vi "Inficon Controller - Main.vi"() -> ()   [LabVIEW 2014]
uses:
  Typedef/Inficon - States.ctl
  Typedef/Inficon - Evaporator parameters.ctl
panel:
  in  "Tab Control":T1(tab)
  in  "Reset":bool
  in  "Run process":bool
  in  "Test Connection":bool
  in  "Set parameters":bool
  in  "Final Thickness":dbl caption="Final Thickness [kÅ]" min=0.0 max=999.0 step=0.001 format="%.;%.3f"
  in  "Exit":bool
  in  "Select Material":u16(ring) items=["None", "Al (Alluminio) - Rotazione", "Al (Alluminio) - Fisso", "Ag (Argento) - Fisso", "Au (Oro) - Rotazione", "Au (Oro) - Fisso", "In (Indio) - Rotazione", "In (Indio) - Fisso", "Cr (Cromo) - Rotazione", "Cr (Cromo) - Fisso", "Cu (Rame) - Rotazione", "Cu (Rame) - Fisso", "Costantana (Cu 55% ; Ni 45%) - Fisso", "Ge (Germanio) - Fisso", "Mo (Molibdeno) - Rotazione", "Mo (Molibdeno) - Fisso", "Pd (Palladio) - Fisso"]
  in  "Deposition Rate":dbl caption="Deposition Rate [Å/s]" min=0.0 max=999.9 step=0.1 format="%.;%.1f"
  in  "Max Power":dbl=0.1 min=0.0 max=100.0 step=0.1 format="%.;%.1f"
  out "Thickness":dbl
  out "Dep rate":dbl
  out "Power":dbl
  in  "Generate XML":bool
  in  "Evap params":T2={"Rise Time 1 [mm:ss]"=0.0, "Soak Power 1 [%]"=0.0, "Soak Time 1 [mm:ss]"=0.0, "Rise Time 2 [mm:ss]"=0.0, "Soak Power 2 [%]"=0.0, "Soak Time 2 [mm:ss]"=0.0, "Shutter Delay"=enum."No", "New Rate"=0.0, "Rate Ramp Time [mm:ss]"=0.0, "Idle Ramp [mm:ss]"=0.0, "Idle Power [%]"=0.0, "Time Power"=enum."No", "Xtal Switch S"=0, "Xtal Switch Q"=0, "Tool Factor 1"=10.0, "Tool Factor 2"=10.0, "Deposition Rate [Å/s]"=0.0, "Final Thickness [kÅ]"=0.0, "Thickness Spt [kÅ]"=0.0, "Density [g/cm3]"=0.5, "Z-Ratio"=0.1, "Sensor"=1, "Source"=1, "Crucible"=1, "Control Gain [%]"=0.1, "Control TC [s]"=0.1, "Control DT [s] 2"=0.1, "Max Power"=0.1, "Sample"=1, "Hold Time [mm:ss]"=0.0} caption="Evaporator parameters" {"Hold Time [mm:ss]" min=0.0 max=5999.0 format="%<%M:%S>t"; "Sample" max=99 step=1; "Max Power" min=0.0 max=100.0 step=0.1 format="%.;%.1f"; "Control DT [s] 2" min=0.1 max=100.0 step=0.1 format="%.;%.1f"; "Control TC [s]" min=0.1 max=100.0 step=0.1 format="%.;%.1f"; "Control Gain [%]" min=0.01 max=99.99 step=0.01 format="%.;%.3f"; "Crucible" max=8 step=1; "Source" min=1 max=2 step=1; "Sensor" min=1 max=2 step=1; "Z-Ratio" min=0.1 max=9.999 step=0.001 format="%.;%.3f"; "Density [g/cm3]" min=0.5 max=99.99 step=0.01 format="%.;%.2f"; "Thickness Spt [kÅ]" min=0.0 max=999.0 step=0.001 format="%.;%.3f"; "Final Thickness [kÅ]" min=0.0 max=999.0 step=0.001 format="%.;%.3f"; "Deposition Rate [Å/s]" min=0.0 max=999.9 step=0.1 format="%.;%.1f"; "Tool Factor 2" min=10.0 max=500.0 step=0.1 format="%.;%.1f"; "Tool Factor 1" min=10.0 max=500.0 step=0.1 format="%.;%.1f"; "Xtal Switch Q" max=9 step=1; "Xtal Switch S" max=9 step=1; "Idle Power [%]" min=0.0 max=100.0 step=0.1 format="%.;%.1f"; "Idle Ramp [mm:ss]" min=0.0 max=5999.0 format="%<%M:%S>t"; "Rate Ramp Time [mm:ss]" min=0.0 max=5999.0 format="%<%M:%S>t"; "New Rate" min=0.0 max=999.9 step=0.1 format="%.;%.1f"; "Soak Time 2 [mm:ss]" min=0.0 max=5999.0 format="%<%M:%S>t"; "Soak Power 2 [%]" min=0.0 max=100.0 step=0.1 format="%.;%.1f"; "Soak Time 1 [mm:ss]" min=0.0 max=5999.0 format="%<%M:%S>t"; "Rise Time 2 [mm:ss]" min=0.0 max=5999.0 format="%<%M:%S>t"; "Soak Power 1 [%]" min=0.0 max=100.0 step=0.1 format="%.;%.1f"; "Rise Time 1 [mm:ss]" min=0.0 max=5999.0 format="%<%M:%S>t"}
  in  "Metal name":string
  out "Thickness Plot":dbl(graph)
  out "Dep rate Plot":dbl(graph)
  out "Power Plot":dbl(graph)
  # "Real time monitor"
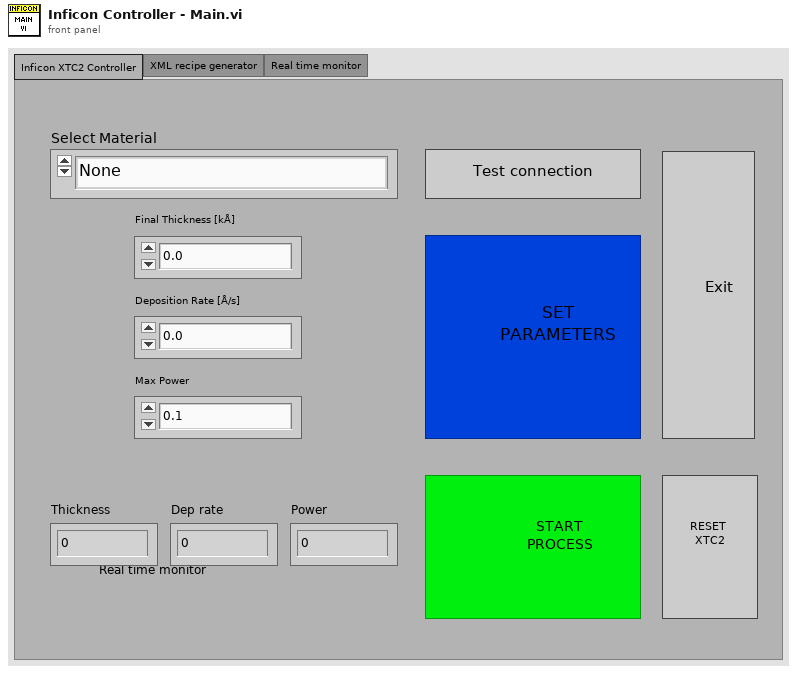
[diagram p1: front panel]
types:
  T1 = enum32{"Inficon XTC2 Controller", "XML recipe generator", "Real time monitor"}
  T2 = typedef "Inficon - Evaporator parameters.ctl" = cluster{"Rise Time 1 [mm:ss]":dbl, "Soak Power 1 [%]":dbl, "Soak Time 1 [mm:ss]":dbl, "Rise Time 2 [mm:ss]":dbl, "Soak Power 2 [%]":dbl, "Soak Time 2 [mm:ss]":dbl, "Shutter Delay":enum16{"No", "Yes"}, "New Rate":dbl, "Rate Ramp Time [mm:ss]":dbl, "Idle Ramp [mm:ss]":dbl, "Idle Power [%]":dbl, "Time Power":enum16{"No", "Yes"}, "Xtal Switch S":u8, "Xtal Switch Q":u8, "Tool Factor 1":dbl, "Tool Factor 2":dbl, "Deposition Rate [Å/s]":dbl, "Final Thickness [kÅ]":dbl, "Thickness Spt [kÅ]":dbl, "Density [g/cm3]":dbl, "Z-Ratio":dbl, "Sensor":u8, "Source":u8, "Crucible":u8, "Control Gain [%]":dbl, "Control TC [s]":dbl, "Control DT [s] 2":dbl, "Max Power":dbl, "Sample":u8, "Hold Time [mm:ss]":dbl}
  T3 = typedef "Inficon - States.ctl" = enum16{"Set Parameters", "Test connection", "Generate XML", "Check for Error", "Set Max Power", "Set Deposition rate", "Read RT parameters", "Start/Stop process", "Reset XTC2", "Exit"}
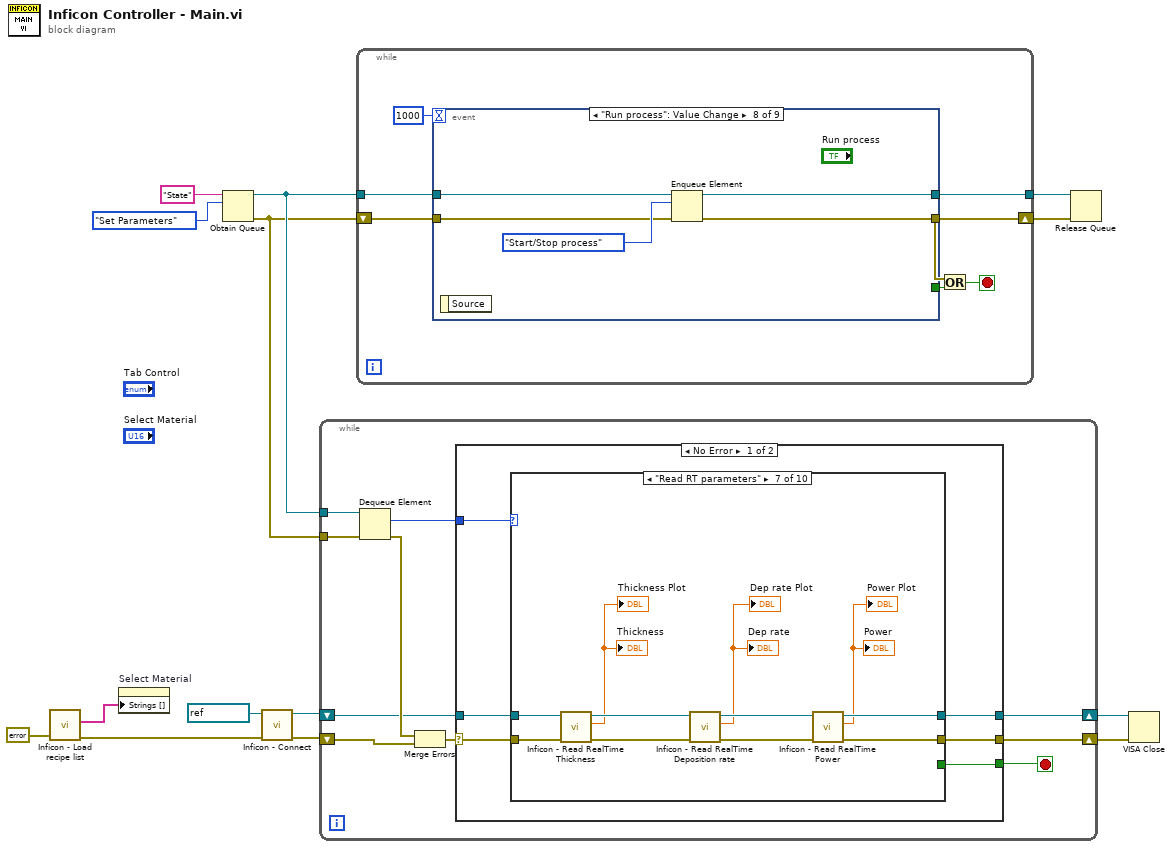
[diagram p0: block diagram]
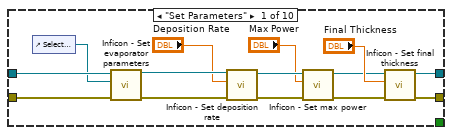
[diagram p2: hidden frame]
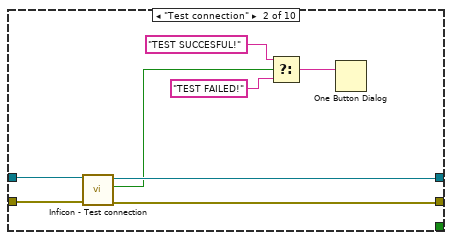
[diagram p3: hidden frame]
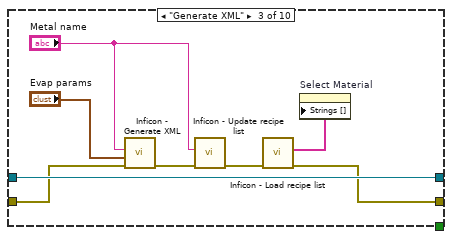
[diagram p4: hidden frame]
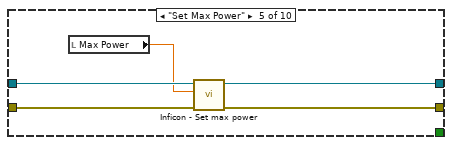
[diagram p6: hidden frame]
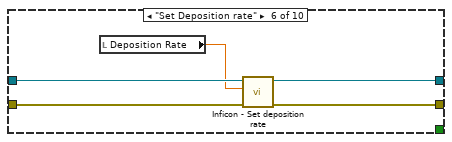
[diagram p7: hidden frame]
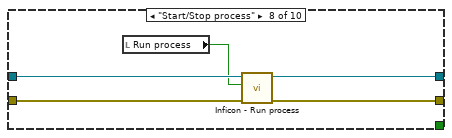
[diagram p8: hidden frame]
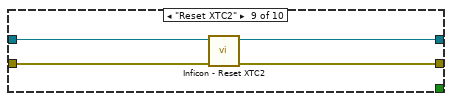
[diagram p9: hidden frame]
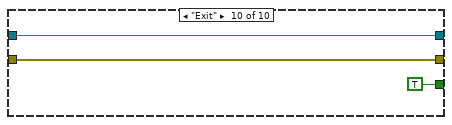
[diagram p10: hidden frame]
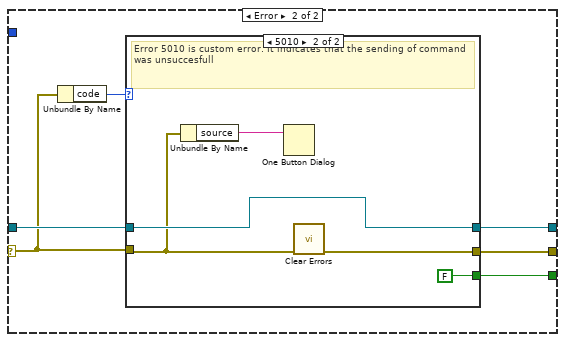
[diagram p11: hidden frame]
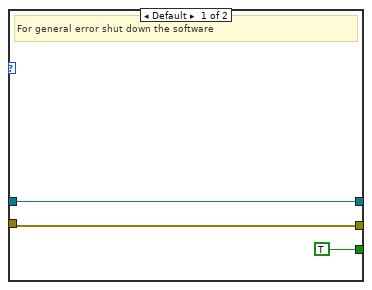
[diagram p12: hidden frame]
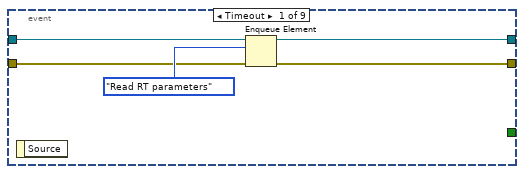
[diagram p13: hidden frame]
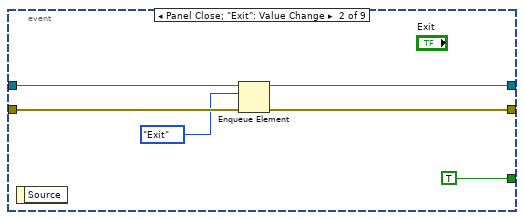
[diagram p14: hidden frame]
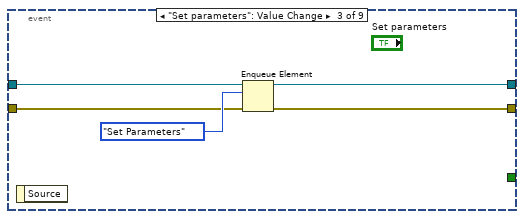
[diagram p15: hidden frame]
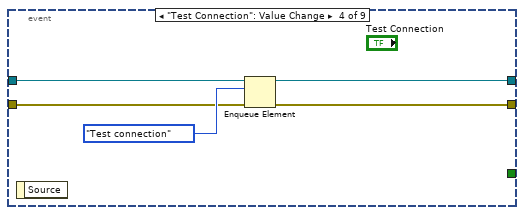
[diagram p16: hidden frame]
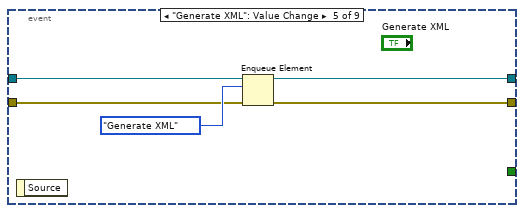
[diagram p17: hidden frame]
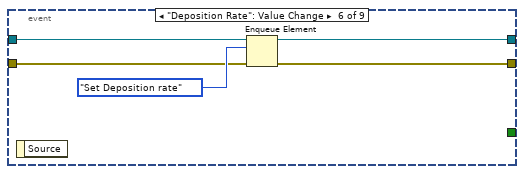
[diagram p18: hidden frame]
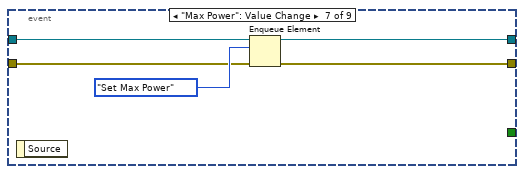
[diagram p19: hidden frame]
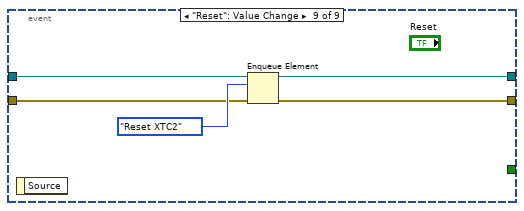
[diagram p20: hidden frame]
diagram:
  n1 = call "Inficon - Load recipe list.vi"("Error In"=errorcluster {"status"=FALSE, "code"=0, "source"=""} ("error out")) -> ("Error Out"=w1:errorcluster, "recipe list"=w5:string[])  [unwired: 9 in]
  n2 = property on="Select Material" class="Ring (strict)"("Strings []"=w5) -> ()  [unwired: 2 in, 2 out]
  n3 = Obtain Queue(name (unnamed)="State", element data type=Inficon_-_States."Set Parameters") -> (queue out=w11:refnum<queue>, error out=w10:errorcluster)  [unwired: 3 in, 1 out]
  n4 = call "Inficon - Connect.vi"("Error In"=w1, "COM in"=refnum<visa-resource-name> "COM5") -> ("Error Out"=w2:errorcluster, "COM out"=w3:refnum<visa-resource-name>)  [unwired: 8 in]
  n5 = while {
    tunnel: w11 -> [w23]
    tunnel: w10 -> [w22]
    shift-right: [w21] -> w8
    shift-left: w2 -> [w19]
    shift-right: [w17] -> w7
    shift-left: w3 -> [w16]
    stop <- w15 stop-if-true
    n6 = Dequeue Element(queue=w23, error in (no error)=w22) -> (element=w24:T3, error out=w18:errorcluster)  [unwired: 1 in, 2 out]
    n7 = Merge Errors(w18, w19) -> (w20:errorcluster)
    n8 = case shown="No Error" w20 {
      selector: w20 -> [w28 w97]
      tunnel: w24 -> [w30 _]
      tunnel: [w25 w100] -> w15
      tunnel: [w29 w96] -> w21
      tunnel: [w27 w99] -> w17
      tunnel: w16 -> [w26 w98]
      frame No Error {
        n9 = case shown="\"Read RT parameters\"" w30 {
          tunnel: [w41 w49 w58 w61 w65 w70 w79 w87 w91 w95] -> w29
          tunnel: w28 -> [w44 w51 w56 w61 w66 w71 w82 w88 w92 w95]
          tunnel: [w42 w50 w60 w62 w64 w69 w76 w85 w89 w94] -> w27
          tunnel: w26 -> [w43 w52 w60 w62 w67 w72 w83 w86 w90 w94]
          tunnel: [_ _ _ _ _ _ _ _ _ TRUE] -> w25
          frame "Set Parameters" {
            n10 = control-ref of="Select Material"() -> (w39:refnum<vi>)
            n11 = call "Inficon - Set evaporator parameters.vi"("Error In"=w44, "Material refnum"=w39, "COM in"=w43) -> ("Error Out"=w33:errorcluster, "COM out"=w38:refnum<visa-resource-name>)  [unwired: 7 in]
            n12 = call "Inficon - Set deposition rate.vi"("Error In"=w33, "Deposition Rate"="Deposition Rate", "COM in"=w38) -> ("Error Out"=w34:errorcluster, "COM out"=w37:refnum<visa-resource-name>)  [unwired: 7 in]
            n13 = call "Inficon - Set max power.vi"("Error In"=w34, "Max Power"="Max Power", "COM in"=w37) -> ("Error Out"=w35:errorcluster, "COM out"=w36:refnum<visa-resource-name>)  [unwired: 7 in]
            n14 = call "Inficon - Set final thickness.vi"("Error In"=w35, "Final Thickness"="Final Thickness", "COM in"=w36) -> ("Error Out"=w41:errorcluster, "COM out"=w42:refnum<visa-resource-name>)  [unwired: 7 in]
          }
          frame "Test connection" {
            n15 = call "Inficon - Test connection.vi"("Error In"=w51, "COM in"=w52) -> ("Error Out"=w49:errorcluster, "Success?"=w48:bool, "COM out"=w50:refnum<visa-resource-name>)  [unwired: 7 in]
            n16 = Select(t="TEST SUCCESFUL!" ("message"), s=w48, f="TEST FAILED!" ("message")) -> (s? t:f=w45:string)
            n17 = One Button Dialog(message=w45) -> ()  [unwired: 1 in, 1 out]
          }
          frame "Generate XML" {
            n18 = call "Inficon - Generate XML.vi"("Error In"=w56, "Evaporator parameters"="Evap params", "Metal name"="Metal name") -> ("Error Out"=w55:errorcluster)  [unwired: 8 in]
            n19 = call "Inficon - Update recipe list.vi"("Error In"=w55, "Metal name"="Metal name") -> ("Error Out"=w54:errorcluster)  [unwired: 9 in]
            n20 = call "Inficon - Load recipe list.vi"("Error In"=w54) -> ("Error Out"=w58:errorcluster, "recipe list"=w59:string[])  [unwired: 9 in]
            n21 = property on="Select Material" class="Ring (strict)"("Strings []"=w59) -> ()  [unwired: 2 in, 2 out]
          }
          frame "Check for Error" {
          }
          frame "Set Max Power" {
            n22 = local read "Max Power"() -> (w63:dbl)
            n23 = call "Inficon - Set max power.vi"("Error In"=w66, "Max Power"=w63, "COM in"=w67) -> ("Error Out"=w65:errorcluster, "COM out"=w64:refnum<visa-resource-name>)  [unwired: 7 in]
          }
          frame "Set Deposition rate" {
            n24 = local read "Deposition Rate"() -> (w68:dbl)
            n25 = call "Inficon - Set deposition rate.vi"("Error In"=w71, "Deposition Rate"=w68, "COM in"=w72) -> ("Error Out"=w70:errorcluster, "COM out"=w69:refnum<visa-resource-name>)  [unwired: 7 in]
          }
          frame "Read RT parameters" {
            n26 = call "Inficon - Read RealTime Thickness.vi"("Error In"=w82, "VISA in"=w83) -> ("Error Out"=w81:errorcluster, "RT Thickness"=→"Thickness" →"Thickness Plot":dbl, "VISA out"=w78:refnum<visa-resource-name>)  [unwired: 6 in, 1 out]
            n27 = call "Inficon - Read RealTime Deposition rate.vi"("Error In"=w81, "VISA in"=w78) -> ("Error Out"=w80:errorcluster, "RT Dep rate"=→"Dep rate" →"Dep rate Plot":dbl, "VISA out"=w77:refnum<visa-resource-name>)  [unwired: 6 in, 1 out]
            n28 = call "Inficon - Read RealTime Power.vi"("Error In"=w80, "VISA in"=w77) -> ("Error Out"=w79:errorcluster, "RT Power"=→"Power" →"Power Plot":dbl, "VISA out"=w76:refnum<visa-resource-name>)  [unwired: 6 in, 1 out]
          }
          frame "Start/Stop process" {
            n29 = local read "Run process"() -> (w84:bool)
            n30 = call "Inficon - Run process.vi"("Error In"=w88, "Run process"=w84, "COM port in"=w86) -> ("Error Out"=w87:errorcluster, "COM port out"=w85:refnum<visa-resource-name>)  [unwired: 7 in]
          }
          frame "Reset XTC2" {
            n31 = call "Inficon - Reset XTC2.vi"("Error In"=w92, "COM port in"=w90) -> ("Error Out"=w91:errorcluster, "COM port out"=w89:refnum<visa-resource-name>)  [unwired: 8 in]
          }
          frame "Exit" {
          }
        }
      }
      frame Error {
        n32 = Unbundle By Name(w97) -> ("code"=w101:i32)
        n33 = case shown="5010" w101 {
          tunnel: [TRUE FALSE] -> w100
          tunnel: [w104 w108] -> w99
          tunnel: w98 -> [w104 w108]
          tunnel: [w103 w107] -> w96
          tunnel: w97 -> [w103 w106]
          frame Default {
            # "For general error shut down the software"
          }
          frame 5010 {
            # "Error 5010 is custom error. It indicates that the sending of command was unsuccesfull"
            n34 = Unbundle By Name(w106) -> ("source"=w105:string)
            n35 = One Button Dialog(message=w105) -> ()  [unwired: 1 in, 1 out]
            n36 = call <vilib>:"Clear Errors.vi"("error in (no error)"=w106) -> ("error out"=w107:errorcluster)  [unwired: 5 in, 1 out]
          }
        }
      }
    }
  }
  n37 = while {
    tunnel: w11 -> [w116]
    tunnel: [w115] -> w14
    shift-right: [w111] -> w13
    shift-left: w10 -> [w114]
    stop <- w113 stop-if-true
    n38 = event shown="[7] \"Run process\": Value Change" {
      selector: _ -> [_ _ _ _ _ _ _ _ _]
      dyn-events: _ -> [_ _ _ _ _ _ _ _ _]
      timeout: 1000 -> [_ _ _ _ _ _ _ _ _]
      tunnel: [w117 w125 w128 w133 w138 w143 w148 w153 w158] -> w115
      tunnel: w116 -> [w120 w126 w131 w136 w141 w146 w151 w156 w161]
      tunnel: w114 -> [w119 w124 w130 w135 w140 w145 w150 w155 w160]
      tunnel: [w118 w123 w129 w134 w139 w144 w149 w154 w159] -> w111
      tunnel: [_ TRUE _ _ _ _ _ _ _] -> w112
      event Timeout {
        n39 = event-data() -> ()  [unwired: 1 in, 1 out]
        n40 = Enqueue Element(queue=w120, element=Inficon_-_States."Read RT parameters", error in (no error)=w119) -> (queue out=w117:refnum<queue>, error out=w118:errorcluster)  [unwired: 1 in, 1 out]
      }
      event Panel Close; "Exit": Value Change {
        n41 = event-data() -> ()  [unwired: 1 in, 1 out]
        n42 = Enqueue Element(queue=w126, element=Inficon_-_States."Exit", error in (no error)=w124) -> (queue out=w125:refnum<queue>, error out=w123:errorcluster)  [unwired: 1 in, 1 out]
      }
      event "Set parameters": Value Change {
        n43 = event-data() -> ()  [unwired: 1 in, 1 out]
        n44 = Enqueue Element(queue=w131, element=Inficon_-_States."Set Parameters", error in (no error)=w130) -> (queue out=w128:refnum<queue>, error out=w129:errorcluster)  [unwired: 1 in, 1 out]
      }
      event "Test Connection": Value Change {
        n45 = event-data() -> ()  [unwired: 1 in, 1 out]
        n46 = Enqueue Element(queue=w136, element=Inficon_-_States."Test connection", error in (no error)=w135) -> (queue out=w133:refnum<queue>, error out=w134:errorcluster)  [unwired: 1 in, 1 out]
      }
      event "Generate XML": Value Change {
        n47 = event-data() -> ()  [unwired: 1 in, 1 out]
        n48 = Enqueue Element(queue=w141, element=Inficon_-_States."Generate XML", error in (no error)=w140) -> (queue out=w138:refnum<queue>, error out=w139:errorcluster)  [unwired: 1 in, 1 out]
      }
      event "Deposition Rate": Value Change {
        n49 = event-data() -> ()  [unwired: 1 in, 1 out]
        n50 = Enqueue Element(queue=w146, element=Inficon_-_States."Set Deposition rate", error in (no error)=w145) -> (queue out=w143:refnum<queue>, error out=w144:errorcluster)  [unwired: 1 in, 1 out]
      }
      event "Max Power": Value Change {
        n51 = event-data() -> ()  [unwired: 1 in, 1 out]
        n52 = Enqueue Element(queue=w151, element=Inficon_-_States."Set Max Power", error in (no error)=w150) -> (queue out=w148:refnum<queue>, error out=w149:errorcluster)  [unwired: 1 in, 1 out]
      }
      event "Run process": Value Change {
        n53 = event-data() -> ()  [unwired: 1 in, 1 out]
        n54 = Enqueue Element(queue=w156, element=Inficon_-_States."Start/Stop process", error in (no error)=w155) -> (queue out=w153:refnum<queue>, error out=w154:errorcluster)  [unwired: 1 in, 1 out]
      }
      event "Reset": Value Change {
        n55 = event-data() -> ()  [unwired: 1 in, 1 out]
        n56 = Enqueue Element(queue=w161, element=Inficon_-_States."Reset XTC2", error in (no error)=w160) -> (queue out=w158:refnum<queue>, error out=w159:errorcluster)  [unwired: 1 in, 1 out]
      }
    }
    n57 = Or(x=w111, y=w112) -> (x .or. y?=w113:bool)
  }
  n58 = Release Queue(queue=w14, error in (no error)=w13) -> ()  [unwired: 1 in, 3 out]
  n59 = VISA Close(VISA resource name=w7, error in (no error)=w8) -> ()  [unwired: 1 out]
